vi "valueToElement.vi"(1 "variant":variant) -> (0 "element":T1)   [LabVIEW 2015]
uses:
  <vilib>/userdefined/High Color/IMAQdx.ctl
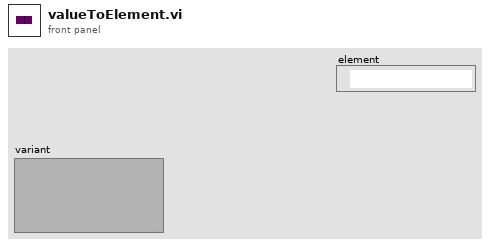
[diagram p1: front panel]
types:
  T1 = typedef "IMAQdx.ctl" = refnum<k21>
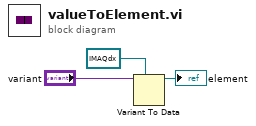
[diagram p0: block diagram]
diagram:
  n1 = Variant To Data(type=T1 refnum ("element"), Variant="variant") -> (data=→"element":T1)  [unwired: 1 in, 1 out]
